vi "boundary (SubVI).vi"(11 "Numeric in":dbl) -> (3 "Numeric out":dbl)   [LabVIEW 2018]
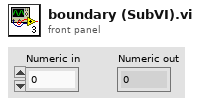
[diagram p1: front panel]
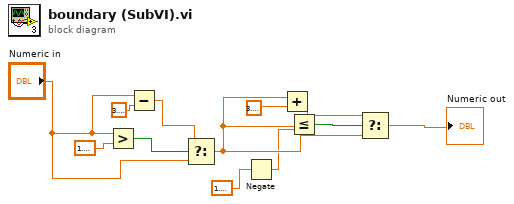
[diagram p0: block diagram]
diagram:
  n1 = Greater?(x="Numeric in", y=1.5707963267948966) -> (0:w5:bool)
  n2 = Subtract(x="Numeric in", y=3.141592653589793) -> (x-y=w7:dbl)
  n3 = Select(t=w7, s=w5, f="Numeric in") -> (s? t:f=w10:dbl)
  n4 = Negate(x=1.5707963267948966) -> (-x=w2:dbl)
  n5 = Add(x=w10, y=3.141592653589793) -> (x+y=w9:dbl)
  n6 = Less Or Equal?(x=w10, y=w2) -> (x <= y?=w8:bool)
  n7 = Select(t=w9, s=w8, f=w10) -> (s? t:f=→"Numeric out":dbl)
